vi "bumper c.vi"() -> ()   [LabVIEW 2013]
uses:
  <vilib>/NXT/Block Support/NXT_InputPort.ctl
  <vilib>/NXT/Block Support/NXT_MessageMailbox.ctl
  <vilib>/NXT/Subs/MotorOutput.ctl
  <vilib>/NXT/Block Support/NXT_OutputPort.ctl
  <vilib>/NXT/Dual Mode Library/Sound/Tone.vi
  <vilib>/NXT/Dual Mode Library/Sound/PlayRedPianoFile.vi
  <vilib>/NXT/NXTIO Xnodes/NXTIONodeSubVIs/NXTStopMotors.vi
  <vilib>/NXT/NXTIO Xnodes/AddressXNode/NXTIOAddress.xnode
  <vilib>/NXT/NXTIO Xnodes/NXTIOXNode/NXTIO.xnode
  <vilib>/NXT/Subs/LVHSConnector.ctl
  <vilib>/NXT/LegoClasses/BrickReference/BrickReference.lvclass
panel:
  out "touch right":bool
  out "touch left":bool
  in  "threshold steer":dbl=0.2
  out "norm dist":dbl
  out "right dist":i16
  out "left dist":i16
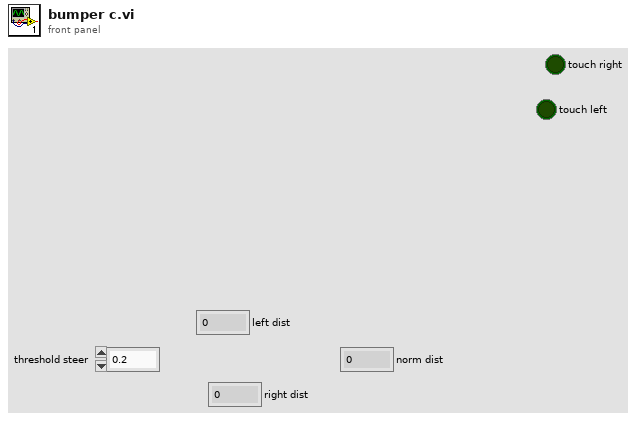
[diagram p1: front panel]
types:
  T1 = typedef "NXT_OutputPort.ctl" = u8
  T2 = typedef "NXT_MessageMailbox.ctl" = u8
  T3 = typedef "NXT_InputPort.ctl" = u32
  T4 = typedef "LVHSConnector.ctl" = refnum<class "BrickReference.lvclass">
  T5 = typedef "MotorOutput.ctl" = u8
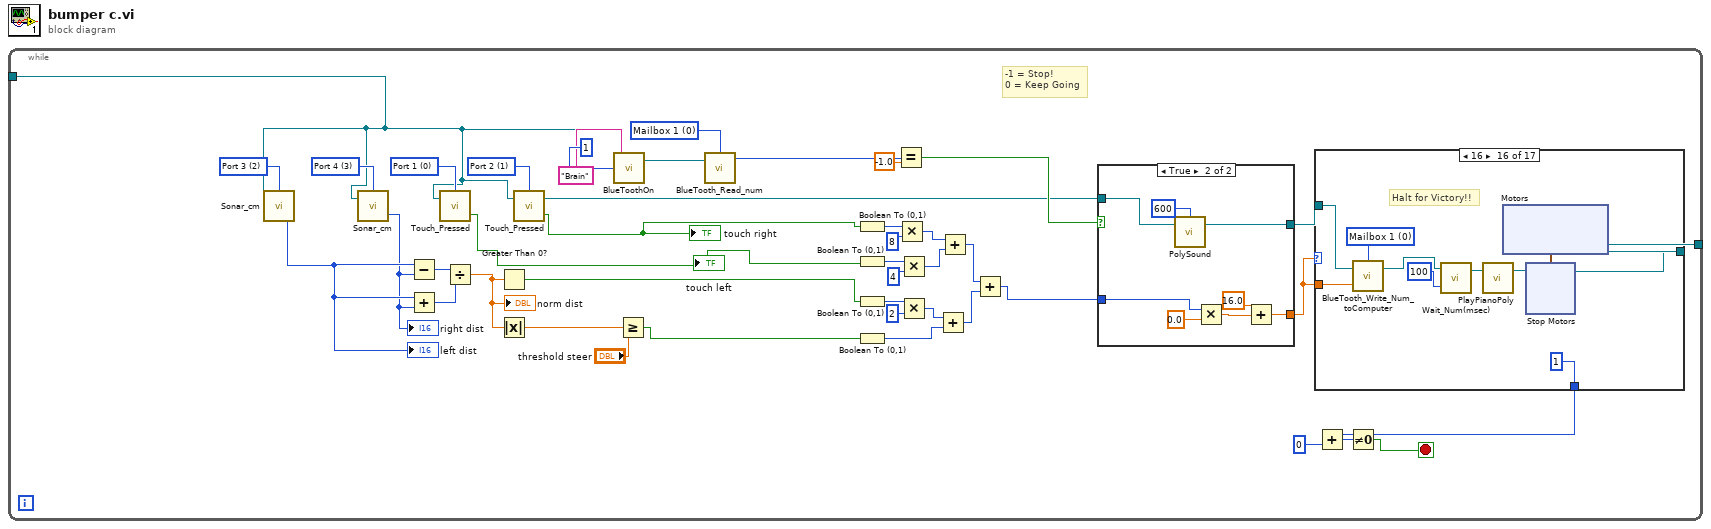
[diagram p0: block diagram]
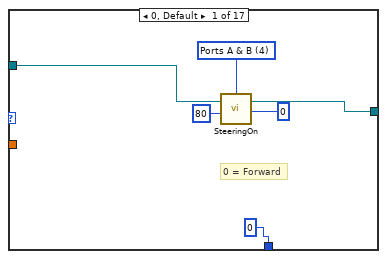
[diagram p3: hidden frame]
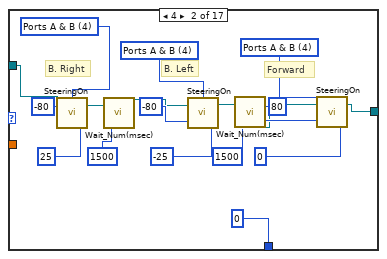
[diagram p4: hidden frame]
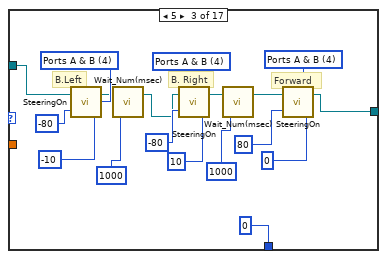
[diagram p5: hidden frame]
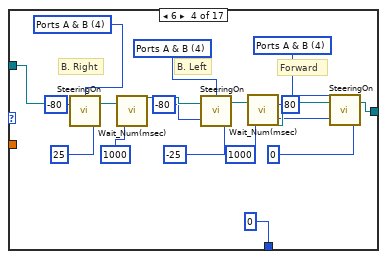
[diagram p6: hidden frame]
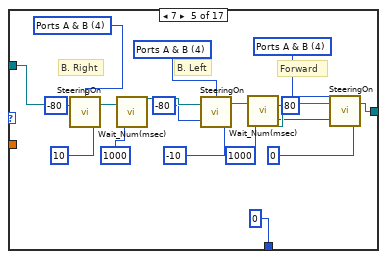
[diagram p7: hidden frame]
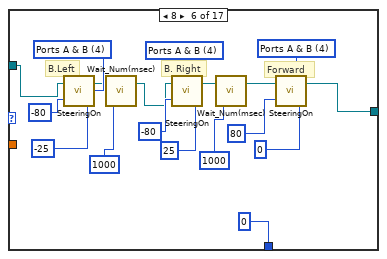
[diagram p8: hidden frame]
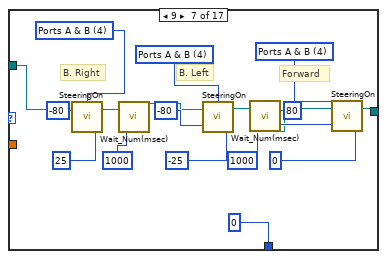
[diagram p9: hidden frame]
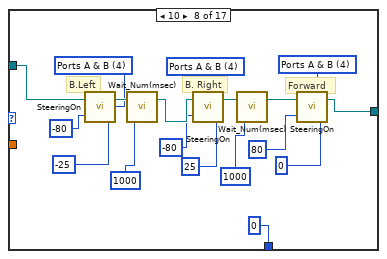
[diagram p10: hidden frame]
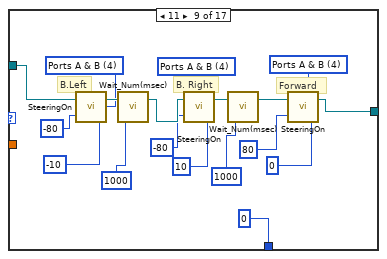
[diagram p11: hidden frame]
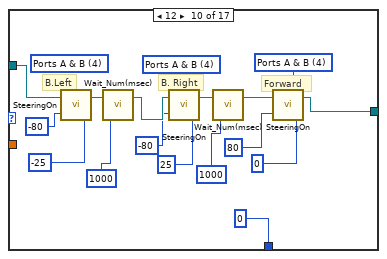
[diagram p12: hidden frame]
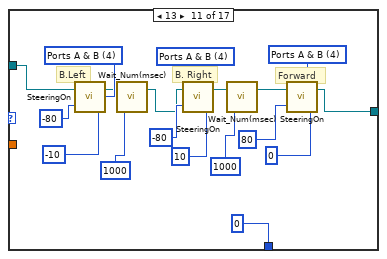
[diagram p13: hidden frame]
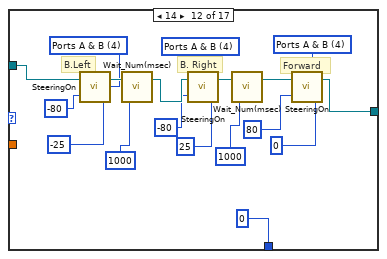
[diagram p14: hidden frame]
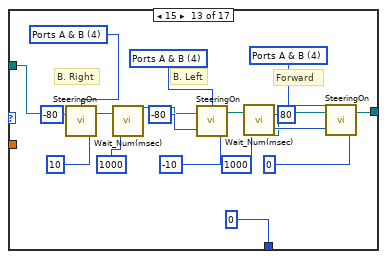
[diagram p15: hidden frame]
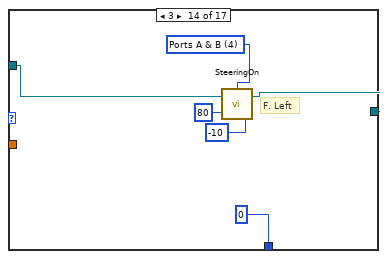
[diagram p16: hidden frame]
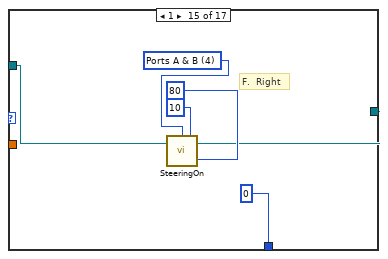
[diagram p17: hidden frame]
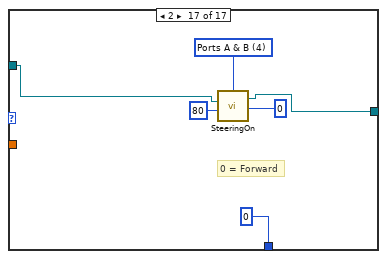
[diagram p18: hidden frame]
diagram:
  n1 = while {
    tunnel: [w15] -> _
    tunnel: [w12] -> _
    stop <- w5 stop-if-true
    w13 = T2 0 items=["Mailbox 1", "Mailbox 2", "Mailbox 3", "Mailbox 4", "Mailbox 5", "Mailbox 6", "Mailbox 7", "Mailbox 8", "Mailbox 9", "Mailbox 10"] ("Mailbox")
    w34 = T3 1 items=["Port 1", "Port 2", "Port 3", "Port 4"] ("Port (Port 1)")
    w35 = T3 0 items=["Port 1", "Port 2", "Port 3", "Port 4"] ("Port (Port 1)")
    w43 = T3 3 items=["Port 1", "Port 2", "Port 3", "Port 4"] ("Port (Port 4)")
    w44 = T3 2 items=["Port 1", "Port 2", "Port 3", "Port 4"] ("Port (Port 4)")
    # "-1 = Stop!\n0 = Keep Going"
    n2 = call <vilib>:"Sonar_cm.vi"("Port (Port 4)"=w44) -> ("Distance (cm)"=w42:i16, "NXT/EV3"=w15:T4)  [unwired: 2 in]
    "left dist" <- w42
    n3 = call <vilib>:"Sonar_cm.vi"("NXT/EV3"=w15, "Port (Port 4)"=w43) -> ("Distance (cm)"=w41:i16)  [unwired: 1 in, 1 out]
    "right dist" <- w41
    n4 = Subtract(x=w42, y=w41) -> (x-y=w40:i16)
    n5 = Add(x=w42, y=w41) -> (x+y=w39:i16)
    n6 = call <vilib>:"Touch_Pressed.vi"("NXT/EV3"=w15, "Port (Port 1)"=w35) -> ("Yes / No"=w21:bool)  [unwired: 1 in, 1 out]
    "touch left" <- w21
    n7 = Divide(x=w40, y=w39) -> (x/y=w36:dbl)
    "norm dist" <- w36
    n8 = Greater Than 0?(x=w36) -> (x > 0?=w19:bool)
    n9 = Absolute Value(x=w36) -> (abs(x)=w38:dbl)
    n10 = call <vilib>:"Touch_Pressed.vi"("NXT/EV3"=w15, "Port (Port 1)"=w34) -> ("Yes / No"=w20:bool, "NXT/EV3"=w3:T4)  [unwired: 1 in]
    "touch right" <- w20
    n11 = call "BlueToothOn.vi"("NXT/EV3"=w15, "Connection"=u8 1, "Partner Name"="Brain") -> ("NXT/EV3 2"=w14:T4)  [unwired: 3 out]
    n12 = Greater Or Equal?(x=w38, y="threshold steer") -> (x >= y?=w18:bool)
    n13 = call <vilib>:"BlueTooth_Read_num.vi"("NXT/EV3"=w14, "Mailbox"=w13) -> ("Message"=w10:i32)  [unwired: 1 in, 1 out]
    n14 = Boolean To (0,1)(Boolean=w20) -> (0, 1=w29:i16)
    n15 = Boolean To (0,1)(Boolean=w21) -> (0, 1=w28:i16)
    n16 = Boolean To (0,1)(Boolean=w19) -> (0, 1=w33:i16)
    n17 = Boolean To (0,1)(Boolean=w18) -> (0, 1=w23:i16)
    n18 = Equal?(x=w10, y=-1.0) -> (x = y?=w9:bool)
    n19 = Multiply(x=w29, y=i16 8) -> (x*y=w26:i16)
    n20 = Multiply(x=w28, y=i16 4) -> (x*y=w25:i16)
    n21 = Multiply(x=w33, y=i16 2) -> (x*y=w24:i16)
    n22 = Add(x=w24, y=w23) -> (x+y=w22:i16)
    n23 = Add(x=w26, y=w25) -> (x+y=w27:i16)
    n24 = Add(x=w27, y=w22) -> (x+y=w4:i16)
    n25 = case shown="True" w9 {
      tunnel: w4 -> [w46 w52]
      tunnel: [w46 w47] -> w1
      tunnel: w3 -> [w45 w51]
      tunnel: [w45 w50] -> w2
      frame False {
      }
      frame True {
        n26 = call-poly <vilib>:"PolySound.vi"("NXT/EV3"=w51, "Tone (440 Hz)"=u16 600) -> ("NXT/EV3"=w50:T4)  [unwired: 2 in]
        n27 = Multiply(x=w52, y=0.0) -> (x*y=w49:dbl)
        n28 = Add(x=16.0, y=w49) -> (x+y=w47:dbl)
      }
    }
    n29 = case shown="16" w1 {
      tunnel: w2 -> [w58 w72 w81 w99 w117 w144 w153 w171 w189 w207 w224 w242 w261 w279 w285 w291 w307]
      tunnel: [w57 w71 w80 w98 w116 w143 w152 w170 w188 w206 w223 w241 w260 w278 w284 w294 w306] -> w12
      tunnel: [0 ("y") 0 ("y") 0 ("y") 0 ("y") 0 ("y") 0 ("y") 0 ("y") 0 ("y") 0 ("y") 0 ("y") 0 ("y") 0 ("y") 0 ("y") 0 ("y") 0 1 0 ("y")] -> w6
      tunnel: w1 -> [_ _ _ _ _ _ _ _ _ _ _ _ _ _ _ w288 _]
      frame 0, Default {
        w56 = T5 4 items=["Port A"=0, "Port B"=1, "Port C"=2, "Ports A & B"=4, "Ports A & C"=5, "Ports B & C"=6, "All Ports"=3] ("Output Ports (A & B) 5")
        # "0 = Forward"
        n30 = call <vilib>:"SteeringOn.vi"("Power (75)"=80, "Steering (100)"=0, "NXT/EV3"=w58, "Output Ports (A & B)"=w56) -> ("NXT/EV3"=w57:T4)
      }
      frame 4 {
        w68 = T5 4 items=["Port A"=0, "Port B"=1, "Port C"=2, "Ports A & B"=4, "Ports A & C"=5, "Ports B & C"=6, "All Ports"=3] ("Output Ports (A & B) 15")
        w69 = T5 4 items=["Port A"=0, "Port B"=1, "Port C"=2, "Ports A & B"=4, "Ports A & C"=5, "Ports B & C"=6, "All Ports"=3] ("Output Port (All Ports) 6")
        w70 = T5 4 items=["Port A"=0, "Port B"=1, "Port C"=2, "Ports A & B"=4, "Ports A & C"=5, "Ports B & C"=6, "All Ports"=3] ("Output Ports (A & B) 16")
        # "Forward"
        # "B. Left"
        # "B. Right"
        n31 = call <vilib>:"SteeringOn.vi"("Power (75)"=-80, "Steering (100)"=25, "NXT/EV3"=w72, "Output Ports (A & B)"=w70) -> ("NXT/EV3"=w67:T4)
        n32 = call <vilib>:"Wait_Num(msec).vi"("Time (100 msec)"=u32 1500, "NXT/EV3"=w67) -> ("NXT/EV3"=w66:T4)  [unwired: 2 in]
        n33 = call <vilib>:"SteeringOn.vi"("Power (75)"=-80, "Steering (100)"=-25, "NXT/EV3"=w66, "Output Ports (A & B)"=w69) -> ("NXT/EV3"=w65:T4)
        n34 = call <vilib>:"Wait_Num(msec).vi"("Time (100 msec)"=u32 1500, "NXT/EV3"=w65) -> ("NXT/EV3"=w64:T4)  [unwired: 2 in]
        n35 = call <vilib>:"SteeringOn.vi"("Power (75)"=80, "Steering (100)"=0, "NXT/EV3"=w64, "Output Ports (A & B)"=w68) -> ("NXT/EV3"=w71:T4)
      }
      frame 5 {
        w88 = T5 4 items=["Port A"=0, "Port B"=1, "Port C"=2, "Ports A & B"=4, "Ports A & C"=5, "Ports B & C"=6, "All Ports"=3] ("Output Ports (A & B) 21")
        w89 = T5 4 items=["Port A"=0, "Port B"=1, "Port C"=2, "Ports A & B"=4, "Ports A & C"=5, "Ports B & C"=6, "All Ports"=3] ("Output Port (All Ports) 9")
        w90 = T5 4 items=["Port A"=0, "Port B"=1, "Port C"=2, "Ports A & B"=4, "Ports A & C"=5, "Ports B & C"=6, "All Ports"=3] ("Output Ports (A & B) 22")
        # "Forward"
        # "B. Right"
        # "B.Left"
        n36 = call <vilib>:"SteeringOn.vi"("Power (75)"=-80, "Steering (100)"=-10, "NXT/EV3"=w81, "Output Ports (A & B)"=w90) -> ("NXT/EV3"=w86:T4)
        n37 = call <vilib>:"Wait_Num(msec).vi"("Time (100 msec)"=u32 1000, "NXT/EV3"=w86) -> ("NXT/EV3"=w85:T4)  [unwired: 2 in]
        n38 = call <vilib>:"SteeringOn.vi"("Power (75)"=-80, "Steering (100)"=10, "NXT/EV3"=w85, "Output Ports (A & B)"=w89) -> ("NXT/EV3"=w83:T4)
        n39 = call <vilib>:"Wait_Num(msec).vi"("Time (100 msec)"=u32 1000, "NXT/EV3"=w83) -> ("NXT/EV3"=w82:T4)  [unwired: 2 in]
        n40 = call <vilib>:"SteeringOn.vi"("Power (75)"=80, "Steering (100)"=0, "NXT/EV3"=w82, "Output Ports (A & B)"=w88) -> ("NXT/EV3"=w80:T4)
      }
      frame 6 {
        w108 = T5 4 items=["Port A"=0, "Port B"=1, "Port C"=2, "Ports A & B"=4, "Ports A & C"=5, "Ports B & C"=6, "All Ports"=3] ("Output Ports (A & B) 15")
        w107 = T5 4 items=["Port A"=0, "Port B"=1, "Port C"=2, "Ports A & B"=4, "Ports A & C"=5, "Ports B & C"=6, "All Ports"=3] ("Output Port (All Ports) 6")
        w106 = T5 4 items=["Port A"=0, "Port B"=1, "Port C"=2, "Ports A & B"=4, "Ports A & C"=5, "Ports B & C"=6, "All Ports"=3] ("Output Ports (A & B) 16")
        # "Forward"
        # "B. Left"
        # "B. Right"
        n41 = call <vilib>:"SteeringOn.vi"("Power (75)"=-80, "Steering (100)"=25, "NXT/EV3"=w99, "Output Ports (A & B)"=w106) -> ("NXT/EV3"=w109:T4)
        n42 = call <vilib>:"Wait_Num(msec).vi"("Time (100 msec)"=u32 1000, "NXT/EV3"=w109) -> ("NXT/EV3"=w110:T4)  [unwired: 2 in]
        n43 = call <vilib>:"SteeringOn.vi"("Power (75)"=-80, "Steering (100)"=-25, "NXT/EV3"=w110, "Output Ports (A & B)"=w107) -> ("NXT/EV3"=w111:T4)
        n44 = call <vilib>:"Wait_Num(msec).vi"("Time (100 msec)"=u32 1000, "NXT/EV3"=w111) -> ("NXT/EV3"=w112:T4)  [unwired: 2 in]
        n45 = call <vilib>:"SteeringOn.vi"("Power (75)"=80, "Steering (100)"=0, "NXT/EV3"=w112, "Output Ports (A & B)"=w108) -> ("NXT/EV3"=w98:T4)
      }
      frame 7 {
        w126 = T5 4 items=["Port A"=0, "Port B"=1, "Port C"=2, "Ports A & B"=4, "Ports A & C"=5, "Ports B & C"=6, "All Ports"=3] ("Output Ports (A & B) 15")
        w125 = T5 4 items=["Port A"=0, "Port B"=1, "Port C"=2, "Ports A & B"=4, "Ports A & C"=5, "Ports B & C"=6, "All Ports"=3] ("Output Port (All Ports) 6")
        w124 = T5 4 items=["Port A"=0, "Port B"=1, "Port C"=2, "Ports A & B"=4, "Ports A & C"=5, "Ports B & C"=6, "All Ports"=3] ("Output Ports (A & B) 16")
        # "Forward"
        # "B. Left"
        # "B. Right"
        n46 = call <vilib>:"SteeringOn.vi"("Power (75)"=-80, "Steering (100)"=10, "NXT/EV3"=w117, "Output Ports (A & B)"=w124) -> ("NXT/EV3"=w127:T4)
        n47 = call <vilib>:"Wait_Num(msec).vi"("Time (100 msec)"=u32 1000, "NXT/EV3"=w127) -> ("NXT/EV3"=w128:T4)  [unwired: 2 in]
        n48 = call <vilib>:"SteeringOn.vi"("Power (75)"=-80, "Steering (100)"=-10, "NXT/EV3"=w128, "Output Ports (A & B)"=w125) -> ("NXT/EV3"=w129:T4)
        n49 = call <vilib>:"Wait_Num(msec).vi"("Time (100 msec)"=u32 1000, "NXT/EV3"=w129) -> ("NXT/EV3"=w130:T4)  [unwired: 2 in]
        n50 = call <vilib>:"SteeringOn.vi"("Power (75)"=80, "Steering (100)"=0, "NXT/EV3"=w130, "Output Ports (A & B)"=w126) -> ("NXT/EV3"=w116:T4)
      }
      frame 8 {
        w140 = T5 4 items=["Port A"=0, "Port B"=1, "Port C"=2, "Ports A & B"=4, "Ports A & C"=5, "Ports B & C"=6, "All Ports"=3] ("Output Ports (A & B) 21")
        w141 = T5 4 items=["Port A"=0, "Port B"=1, "Port C"=2, "Ports A & B"=4, "Ports A & C"=5, "Ports B & C"=6, "All Ports"=3] ("Output Port (All Ports) 9")
        w142 = T5 4 items=["Port A"=0, "Port B"=1, "Port C"=2, "Ports A & B"=4, "Ports A & C"=5, "Ports B & C"=6, "All Ports"=3] ("Output Ports (A & B) 22")
        # "Forward"
        # "B. Right"
        # "B.Left"
        n51 = call <vilib>:"SteeringOn.vi"("Power (75)"=-80, "Steering (100)"=-25, "NXT/EV3"=w144, "Output Ports (A & B)"=w142) -> ("NXT/EV3"=w138:T4)
        n52 = call <vilib>:"Wait_Num(msec).vi"("Time (100 msec)"=u32 1000, "NXT/EV3"=w138) -> ("NXT/EV3"=w137:T4)  [unwired: 2 in]
        n53 = call <vilib>:"SteeringOn.vi"("Power (75)"=-80, "Steering (100)"=25, "NXT/EV3"=w137, "Output Ports (A & B)"=w141) -> ("NXT/EV3"=w135:T4)
        n54 = call <vilib>:"Wait_Num(msec).vi"("Time (100 msec)"=u32 1000, "NXT/EV3"=w135) -> ("NXT/EV3"=w134:T4)  [unwired: 2 in]
        n55 = call <vilib>:"SteeringOn.vi"("Power (75)"=80, "Steering (100)"=0, "NXT/EV3"=w134, "Output Ports (A & B)"=w140) -> ("NXT/EV3"=w143:T4)
      }
      frame 9 {
        w160 = T5 4 items=["Port A"=0, "Port B"=1, "Port C"=2, "Ports A & B"=4, "Ports A & C"=5, "Ports B & C"=6, "All Ports"=3] ("Output Ports (A & B) 15")
        w161 = T5 4 items=["Port A"=0, "Port B"=1, "Port C"=2, "Ports A & B"=4, "Ports A & C"=5, "Ports B & C"=6, "All Ports"=3] ("Output Port (All Ports) 6")
        w162 = T5 4 items=["Port A"=0, "Port B"=1, "Port C"=2, "Ports A & B"=4, "Ports A & C"=5, "Ports B & C"=6, "All Ports"=3] ("Output Ports (A & B) 16")
        # "Forward"
        # "B. Left"
        # "B. Right"
        n56 = call <vilib>:"SteeringOn.vi"("Power (75)"=-80, "Steering (100)"=25, "NXT/EV3"=w153, "Output Ports (A & B)"=w162) -> ("NXT/EV3"=w159:T4)
        n57 = call <vilib>:"Wait_Num(msec).vi"("Time (100 msec)"=u32 1000, "NXT/EV3"=w159) -> ("NXT/EV3"=w158:T4)  [unwired: 2 in]
        n58 = call <vilib>:"SteeringOn.vi"("Power (75)"=-80, "Steering (100)"=-25, "NXT/EV3"=w158, "Output Ports (A & B)"=w161) -> ("NXT/EV3"=w157:T4)
        n59 = call <vilib>:"Wait_Num(msec).vi"("Time (100 msec)"=u32 1000, "NXT/EV3"=w157) -> ("NXT/EV3"=w156:T4)  [unwired: 2 in]
        n60 = call <vilib>:"SteeringOn.vi"("Power (75)"=80, "Steering (100)"=0, "NXT/EV3"=w156, "Output Ports (A & B)"=w160) -> ("NXT/EV3"=w152:T4)
      }
      frame 10 {
        w180 = T5 4 items=["Port A"=0, "Port B"=1, "Port C"=2, "Ports A & B"=4, "Ports A & C"=5, "Ports B & C"=6, "All Ports"=3] ("Output Ports (A & B) 21")
        w179 = T5 4 items=["Port A"=0, "Port B"=1, "Port C"=2, "Ports A & B"=4, "Ports A & C"=5, "Ports B & C"=6, "All Ports"=3] ("Output Port (All Ports) 9")
        w178 = T5 4 items=["Port A"=0, "Port B"=1, "Port C"=2, "Ports A & B"=4, "Ports A & C"=5, "Ports B & C"=6, "All Ports"=3] ("Output Ports (A & B) 22")
        # "Forward"
        # "B. Right"
        # "B.Left"
        n61 = call <vilib>:"SteeringOn.vi"("Power (75)"=-80, "Steering (100)"=-25, "NXT/EV3"=w171, "Output Ports (A & B)"=w178) -> ("NXT/EV3"=w182:T4)
        n62 = call <vilib>:"Wait_Num(msec).vi"("Time (100 msec)"=u32 1000, "NXT/EV3"=w182) -> ("NXT/EV3"=w183:T4)  [unwired: 2 in]
        n63 = call <vilib>:"SteeringOn.vi"("Power (75)"=-80, "Steering (100)"=25, "NXT/EV3"=w183, "Output Ports (A & B)"=w179) -> ("NXT/EV3"=w185:T4)
        n64 = call <vilib>:"Wait_Num(msec).vi"("Time (100 msec)"=u32 1000, "NXT/EV3"=w185) -> ("NXT/EV3"=w186:T4)  [unwired: 2 in]
        n65 = call <vilib>:"SteeringOn.vi"("Power (75)"=80, "Steering (100)"=0, "NXT/EV3"=w186, "Output Ports (A & B)"=w180) -> ("NXT/EV3"=w170:T4)
      }
      frame 11 {
        w198 = T5 4 items=["Port A"=0, "Port B"=1, "Port C"=2, "Ports A & B"=4, "Ports A & C"=5, "Ports B & C"=6, "All Ports"=3] ("Output Ports (A & B) 21")
        w197 = T5 4 items=["Port A"=0, "Port B"=1, "Port C"=2, "Ports A & B"=4, "Ports A & C"=5, "Ports B & C"=6, "All Ports"=3] ("Output Port (All Ports) 9")
        w196 = T5 4 items=["Port A"=0, "Port B"=1, "Port C"=2, "Ports A & B"=4, "Ports A & C"=5, "Ports B & C"=6, "All Ports"=3] ("Output Ports (A & B) 22")
        # "Forward"
        # "B. Right"
        # "B.Left"
        n66 = call <vilib>:"SteeringOn.vi"("Power (75)"=-80, "Steering (100)"=-10, "NXT/EV3"=w189, "Output Ports (A & B)"=w196) -> ("NXT/EV3"=w200:T4)
        n67 = call <vilib>:"Wait_Num(msec).vi"("Time (100 msec)"=u32 1000, "NXT/EV3"=w200) -> ("NXT/EV3"=w201:T4)  [unwired: 2 in]
        n68 = call <vilib>:"SteeringOn.vi"("Power (75)"=-80, "Steering (100)"=10, "NXT/EV3"=w201, "Output Ports (A & B)"=w197) -> ("NXT/EV3"=w203:T4)
        n69 = call <vilib>:"Wait_Num(msec).vi"("Time (100 msec)"=u32 1000, "NXT/EV3"=w203) -> ("NXT/EV3"=w204:T4)  [unwired: 2 in]
        n70 = call <vilib>:"SteeringOn.vi"("Power (75)"=80, "Steering (100)"=0, "NXT/EV3"=w204, "Output Ports (A & B)"=w198) -> ("NXT/EV3"=w188:T4)
      }
      frame 12 {
        w215 = T5 4 items=["Port A"=0, "Port B"=1, "Port C"=2, "Ports A & B"=4, "Ports A & C"=5, "Ports B & C"=6, "All Ports"=3] ("Output Ports (A & B) 21")
        w214 = T5 4 items=["Port A"=0, "Port B"=1, "Port C"=2, "Ports A & B"=4, "Ports A & C"=5, "Ports B & C"=6, "All Ports"=3] ("Output Port (All Ports) 9")
        (unwired) T5 4 items=["Port A"=0, "Port B"=1, "Port C"=2, "Ports A & B"=4, "Ports A & C"=5, "Ports B & C"=6, "All Ports"=3] ("Output Ports (A & B) 22")
        # "Forward"
        # "B. Right"
        # "B.Left"
        n71 = call <vilib>:"SteeringOn.vi"("Power (75)"=-80, "Steering (100)"=-25, "NXT/EV3"=w207) -> ("NXT/EV3"=w217:T4)  [unwired: 1 in]
        n72 = call <vilib>:"Wait_Num(msec).vi"("Time (100 msec)"=u32 1000, "NXT/EV3"=w217) -> ("NXT/EV3"=w218:T4)  [unwired: 2 in]
        n73 = call <vilib>:"SteeringOn.vi"("Power (75)"=-80, "Steering (100)"=25, "NXT/EV3"=w218, "Output Ports (A & B)"=w214) -> ("NXT/EV3"=w220:T4)
        n74 = call <vilib>:"Wait_Num(msec).vi"("Time (100 msec)"=u32 1000, "NXT/EV3"=w220) -> ("NXT/EV3"=w221:T4)  [unwired: 2 in]
        n75 = call <vilib>:"SteeringOn.vi"("Power (75)"=80, "Steering (100)"=0, "NXT/EV3"=w221, "Output Ports (A & B)"=w215) -> ("NXT/EV3"=w206:T4)
      }
      frame 13 {
        w231 = T5 4 items=["Port A"=0, "Port B"=1, "Port C"=2, "Ports A & B"=4, "Ports A & C"=5, "Ports B & C"=6, "All Ports"=3] ("Output Ports (A & B) 21")
        w232 = T5 4 items=["Port A"=0, "Port B"=1, "Port C"=2, "Ports A & B"=4, "Ports A & C"=5, "Ports B & C"=6, "All Ports"=3] ("Output Port (All Ports) 9")
        w233 = T5 4 items=["Port A"=0, "Port B"=1, "Port C"=2, "Ports A & B"=4, "Ports A & C"=5, "Ports B & C"=6, "All Ports"=3] ("Output Ports (A & B) 22")
        # "Forward"
        # "B. Right"
        # "B.Left"
        n76 = call <vilib>:"SteeringOn.vi"("Power (75)"=-80, "Steering (100)"=-10, "NXT/EV3"=w224, "Output Ports (A & B)"=w233) -> ("NXT/EV3"=w229:T4)
        n77 = call <vilib>:"Wait_Num(msec).vi"("Time (100 msec)"=u32 1000, "NXT/EV3"=w229) -> ("NXT/EV3"=w228:T4)  [unwired: 2 in]
        n78 = call <vilib>:"SteeringOn.vi"("Power (75)"=-80, "Steering (100)"=10, "NXT/EV3"=w228, "Output Ports (A & B)"=w232) -> ("NXT/EV3"=w226:T4)
        n79 = call <vilib>:"Wait_Num(msec).vi"("Time (100 msec)"=u32 1000, "NXT/EV3"=w226) -> ("NXT/EV3"=w225:T4)  [unwired: 2 in]
        n80 = call <vilib>:"SteeringOn.vi"("Power (75)"=80, "Steering (100)"=0, "NXT/EV3"=w225, "Output Ports (A & B)"=w231) -> ("NXT/EV3"=w223:T4)
      }
      frame 14 {
        w251 = T5 4 items=["Port A"=0, "Port B"=1, "Port C"=2, "Ports A & B"=4, "Ports A & C"=5, "Ports B & C"=6, "All Ports"=3] ("Output Ports (A & B) 21")
        w250 = T5 4 items=["Port A"=0, "Port B"=1, "Port C"=2, "Ports A & B"=4, "Ports A & C"=5, "Ports B & C"=6, "All Ports"=3] ("Output Port (All Ports) 9")
        w249 = T5 4 items=["Port A"=0, "Port B"=1, "Port C"=2, "Ports A & B"=4, "Ports A & C"=5, "Ports B & C"=6, "All Ports"=3] ("Output Ports (A & B) 22")
        # "Forward"
        # "B. Right"
        # "B.Left"
        n81 = call <vilib>:"SteeringOn.vi"("Power (75)"=-80, "Steering (100)"=-25, "NXT/EV3"=w242, "Output Ports (A & B)"=w249) -> ("NXT/EV3"=w253:T4)
        n82 = call <vilib>:"Wait_Num(msec).vi"("Time (100 msec)"=u32 1000, "NXT/EV3"=w253) -> ("NXT/EV3"=w254:T4)  [unwired: 2 in]
        n83 = call <vilib>:"SteeringOn.vi"("Power (75)"=-80, "Steering (100)"=25, "NXT/EV3"=w254, "Output Ports (A & B)"=w250) -> ("NXT/EV3"=w256:T4)
        n84 = call <vilib>:"Wait_Num(msec).vi"("Time (100 msec)"=u32 1000, "NXT/EV3"=w256) -> ("NXT/EV3"=w257:T4)  [unwired: 2 in]
        n85 = call <vilib>:"SteeringOn.vi"("Power (75)"=80, "Steering (100)"=0, "NXT/EV3"=w257, "Output Ports (A & B)"=w251) -> ("NXT/EV3"=w241:T4)
      }
      frame 15 {
        w268 = T5 4 items=["Port A"=0, "Port B"=1, "Port C"=2, "Ports A & B"=4, "Ports A & C"=5, "Ports B & C"=6, "All Ports"=3] ("Output Ports (A & B) 15")
        w269 = T5 4 items=["Port A"=0, "Port B"=1, "Port C"=2, "Ports A & B"=4, "Ports A & C"=5, "Ports B & C"=6, "All Ports"=3] ("Output Port (All Ports) 6")
        w259 = T5 4 items=["Port A"=0, "Port B"=1, "Port C"=2, "Ports A & B"=4, "Ports A & C"=5, "Ports B & C"=6, "All Ports"=3] ("Output Ports (A & B) 16")
        # "Forward"
        # "B. Left"
        # "B. Right"
        n86 = call <vilib>:"SteeringOn.vi"("Power (75)"=-80, "Steering (100)"=10, "NXT/EV3"=w261, "Output Ports (A & B)"=w259) -> ("NXT/EV3"=w267:T4)
        n87 = call <vilib>:"Wait_Num(msec).vi"("Time (100 msec)"=u32 1000, "NXT/EV3"=w267) -> ("NXT/EV3"=w266:T4)  [unwired: 2 in]
        n88 = call <vilib>:"SteeringOn.vi"("Power (75)"=-80, "Steering (100)"=-10, "NXT/EV3"=w266, "Output Ports (A & B)"=w269) -> ("NXT/EV3"=w265:T4)
        n89 = call <vilib>:"Wait_Num(msec).vi"("Time (100 msec)"=u32 1000, "NXT/EV3"=w265) -> ("NXT/EV3"=w264:T4)  [unwired: 2 in]
        n90 = call <vilib>:"SteeringOn.vi"("Power (75)"=80, "Steering (100)"=0, "NXT/EV3"=w264, "Output Ports (A & B)"=w268) -> ("NXT/EV3"=w260:T4)
      }
      frame 3 {
        w277 = T5 4 items=["Port A"=0, "Port B"=1, "Port C"=2, "Ports A & B"=4, "Ports A & C"=5, "Ports B & C"=6, "All Ports"=3] ("Output Port (All Ports) 3")
        # "F. Left"
        n91 = call <vilib>:"SteeringOn.vi"("Power (75)"=80, "Steering (100)"=-10, "NXT/EV3"=w279, "Output Ports (A & B)"=w277) -> ("NXT/EV3"=w278:T4)
      }
      frame 1 {
        w283 = T5 4 items=["Port A"=0, "Port B"=1, "Port C"=2, "Ports A & B"=4, "Ports A & C"=5, "Ports B & C"=6, "All Ports"=3] ("Output Ports (A & B) 12")
        # "F.  Right"
        n92 = call <vilib>:"SteeringOn.vi"("Power (75)"=80, "Steering (100)"=10, "NXT/EV3"=w285, "Output Ports (A & B)"=w283) -> ("NXT/EV3"=w284:T4)
      }
      frame 16 {
        w289 = T2 0 items=["Mailbox 1", "Mailbox 2", "Mailbox 3", "Mailbox 4", "Mailbox 5", "Mailbox 6", "Mailbox 7", "Mailbox 8", "Mailbox 9", "Mailbox 10"] ("Mailbox")
        # "Halt for Victory!!"
        n93 = call <vilib>:"BlueTooth_Write_Num_toComputer.vi"("Message in"=w288, "NXT/EV3"=w291, "Mailbox"=w289) -> ("NXT/EV3"=w290:T4)  [unwired: 1 in]
        n94 = call <vilib>:"Wait_Num(msec).vi"("Time (100 msec)"=u32 100, "NXT/EV3"=w290) -> ("NXT/EV3"=w293:T4)  [unwired: 2 in]
        n95 = call-poly <vilib>:"PlayPianoPoly.vi"("NXT/EV3"=w293) -> ("NXT/EV3"=w292:T4)  [unwired: 3 in]
        n96 = xnode "Motors"() -> ("Motor"=w297:cluster{"Port":T1, "Port":T1})
        n97 = xnode "Stop Motors"("Motors"=w297, "NXT/EV3"=w292) -> ("NXT/EV3"=w294:T4)
      }
      frame 2 {
        w305 = T5 4 items=["Port A"=0, "Port B"=1, "Port C"=2, "Ports A & B"=4, "Ports A & C"=5, "Ports B & C"=6, "All Ports"=3] ("Output Ports (A & B) 10")
        # "0 = Forward"
        n98 = call <vilib>:"SteeringOn.vi"("Power (75)"=80, "Steering (100)"=0, "NXT/EV3"=w307, "Output Ports (A & B)"=w305) -> ("NXT/EV3"=w306:T4)
      }
    }
    n99 = Add(x=w6, y=0) -> (x+y=w7:i32)
    n100 = Not Equal To 0?(x=w7) -> (x != 0?=w5:bool)
  }
